vi "SMTP Email Reply To Error.vi"(4 "error in (no error)":errorcluster, 5 "reply string in":string, 6 "reply code in":i32, 7 "smtp session":T1) -> (0 "error out":errorcluster, 1 "duplicate reply string":string, 2 "duplicate reply code":i32, 3 "smtp session out":T1)   [LabVIEW 2011, in "NewNI_SMTPEmail.lvlib"]
doc: "Parses the first three digits from the reply string of SMTP server and sets the error condition in \"error out\" cluster to true if the error code is over 400. In case of error, it also sets the error code field of the cluster to the parsed error code, and source field to the reply string (not including error code)."
uses:
  NewNI_SMTPEmail.lvlib
  SMTP Email Session.ctl
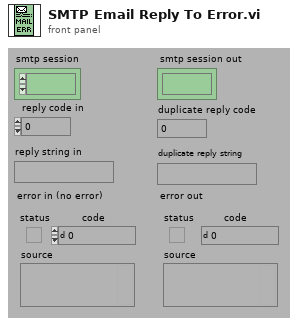
[diagram p1: front panel]
types:
  T1 = typedef "NewNI_SMTPEmail.lvlib/SMTP Email Session.ctl" = refnum<k1>
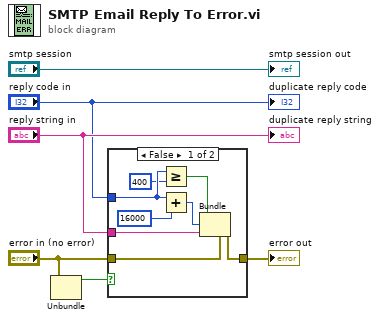
[diagram p0: block diagram]
diagram:
  n1 = Unbundle("error in (no error)") -> ("status"=w1:bool)  [unwired: 2 out]
  n2 = case shown="False" w1 {
    tunnel: "reply code in" -> [w14 _]
    tunnel: [w13 w15] -> w4
    tunnel: "reply string in" -> [w10 _]
    tunnel: "error in (no error)" -> [w9 w15]
    frame False {
      n3 = Greater Or Equal?(x=w14, y=400) -> (x >= y?=w8:bool)
      n4 = Add(x=w14, y=16000) -> (x+y=w12:i32)
      n5 = Bundle(cluster=w9, "status"=w8, "code"=w12, "source"=w10) -> (w13:errorcluster)
    }
    frame True {
    }
  }
  "error out" <- w4
  "duplicate reply code" <- "reply code in"
  "duplicate reply string" <- "reply string in"
  "smtp session out" <- "smtp session"
